vi "Are two within tolerance of each other.vi"(9 "tolerance":dbl, 10 "number 2":dbl, 11 "number":dbl) -> (3 "In range":bool)   [LabVIEW 2020]
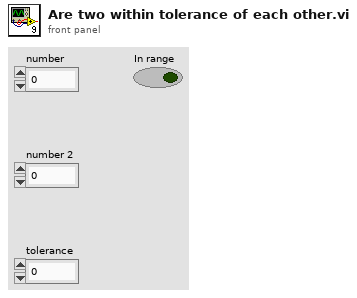
[diagram p1: front panel]
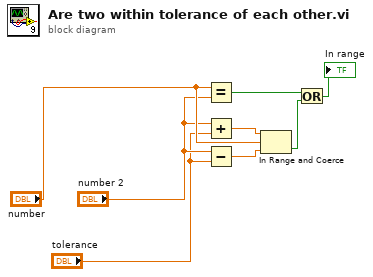
[diagram p0: block diagram]
diagram:
  n1 = Equal?(x="number", y="number 2") -> (x = y?=w2:bool)
  n2 = Add(x="number 2", y="tolerance") -> (x+y=w5:dbl)
  n3 = Subtract(x="number 2", y="tolerance") -> (x-y=w4:dbl)
  n4 = In Range and Coerce(upper limit=w5, x="number", lower limit=w4) -> (In Range?=w3:bool)  [unwired: 1 out]
  n5 = Or(x=w2, y=w3) -> (x .or. y?=→"In range":bool)
